vi "Generador Encendido-Apagado.vi"(8 "error in (no error)":errorcluster, 10 "Estatus del Generador":bool) -> (0 "error out":errorcluster)   [LabVIEW 2020, in "Main.lvlib"]
doc: "Indica a los módulos que escuchan, que el botón de encendido del generado ha sido presionado, contiene el Estatus actual del generador\n_____\nCreated using Delacor QMH Event Scripter 5.0.0.112."
uses:
  Main.lvlib
  Generador Encendido-Apagado Argument--cluster.ctl
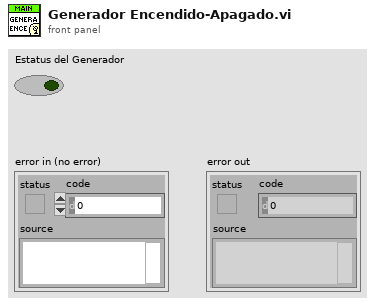
[diagram p1: front panel]
types:
  T1 = typedef "Main.lvlib/Generador Encendido-Apagado Argument--cluster.ctl" = cluster{"Estatus del Generador":bool}
  T2 = typedef "Main.lvlib/Broadcast Events--cluster.ctl" = cluster{"Module Did Init":refnum<user-event>, "Status Updated":refnum<user-event>, "Error Reported":refnum<user-event>, "Module Did Stop":refnum<user-event>, "Update Module Execution Status":refnum<user-event>, "Generador Encendido-Apagado":refnum<user-event>}
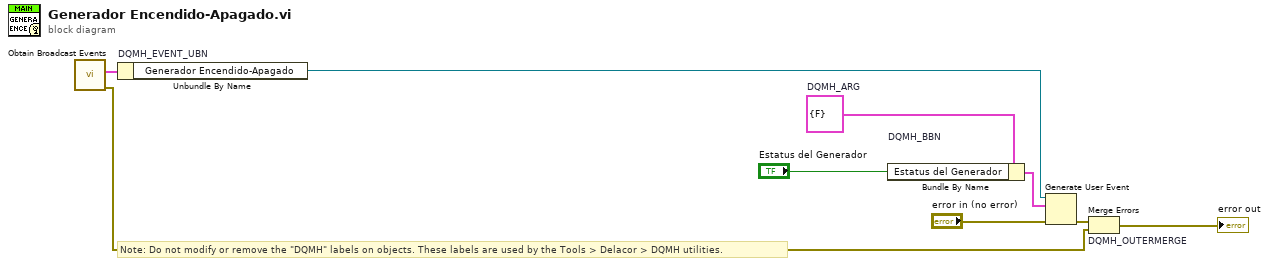
[diagram p0: block diagram]
diagram:
  w4 = T1 {"Estatus del Generador"=FALSE}  # DQMH_ARG
  # "Note: Do not modify or remove the \"DQMH\" labels on objects. These labels are used by the Tools > Delacor > DQMH utilities."
  n1 = call "Obtain Broadcast Events.vi"() -> ("error out"=w2:errorcluster, "Main Broadcast Events"=w1:T2)  [unwired: 10 in]
  n2 = Unbundle By Name "DQMH_EVENT_UBN"(w1) -> ("Generador Encendido-Apagado"=w6:refnum<user-event>)
  n3 = Bundle By Name "DQMH_BBN"(cluster=w4, "Estatus del Generador"="Estatus del Generador") -> (w7:T1)
  n4 = Generate User Event(user event=w6, event data cluster=w7, error in="error in (no error)") -> (error out=w5:errorcluster)  [unwired: 1 in, 1 out]
  n5 = Merge Errors "DQMH_OUTERMERGE"(w5, w2) -> (→"error out":errorcluster)
